vi "KObjTemplate-Factory (by name).vi"(0 "Obj in":refnum<class "KObject.lvclass">, 7 "Class Name":string, 11 "error in (no error)":errorcluster) -> (4 "Obj out":refnum<class "KObject.lvclass">, 15 "error out":errorcluster)   [LabVIEW 2015]
uses:
  KObject Class/KObject.lvclass
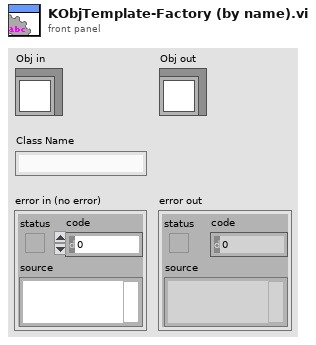
[diagram p1: front panel]
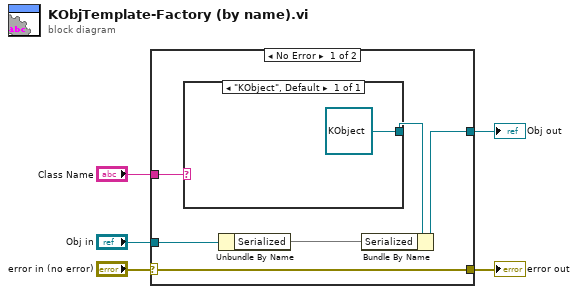
[diagram p0: block diagram]
diagram:
  n1 = case shown="No Error" "error in (no error)" {
    selector: "error in (no error)" -> [w9 w14]
    tunnel: [w9 w14] -> w4
    tunnel: [w7 w13] -> w2
    tunnel: "Obj in" -> [w8 w13]
    tunnel: "Class Name" -> [w10 _]
    frame No Error {
      n2 = case shown="\"KObject\", Default" w10 {
        tunnel: [refnum<class "KObject.lvclass"> refnum ("KObject")] -> w11
        frame "KObject", Default {
        }
      }
      n3 = Unbundle By Name(w8) -> ("Serialized"=w6)
      n4 = Bundle By Name(cluster=w11, "Serialized"=w6) -> (w7:refnum<class "KObject.lvclass">)
    }
    frame Error {
    }
  }
  "error out" <- w4
  "Obj out" <- w2
